vi "Button States Read.vi"(4 "error in (no error)":errorcluster, 6 "Container State":T3, 7 "Display State In":T1={"Buttons Displayed"=0, "Button States"=[], "Button Size"=0, "Button Style"=enum."Classic", "Active Button"=0, "Force Regen?"=FALSE, "Tip String Ref"=refnum}) -> (0 "error out":errorcluster, 2 "Value":bool[](array[boolean]), 3 "Display State Out":T1={"Buttons Displayed"=0, "Button States"=[], "Button Size"=0, "Button Style"=enum."Classic", "Active Button"=0, "Force Regen?"=FALSE, "Tip String Ref"=refnum})   [LabVIEW 2012, in "Toolbar.xctl"]
doc: "Read back which of the current buttons are in the 'on' state."
uses:
  Toolbar.xctl
  <vilib>/_xctls/Container State.ctl
  Toolbar State.ctl
  Button_Class/Button.lvclass
  Button_Class/Type Defs/Button Style.ctl
  Button_Class/Type Defs/Button Status.ctl
  <vilib>/_xctls/XControlSupport.lvlib
panel:
  # "Replace the Value Indicator below with an Indicator of desired type.\nDo not remove this Indicator or the others from the connector pane. \nDo not change the connector pane pattern.\nThe Value Indicator should always be the second terminal from top on the output side in the connector pane."
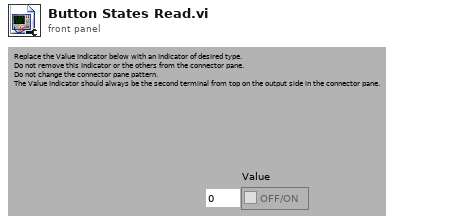
[diagram p1: front panel]
types:
  T1 = typedef "Toolbar.xctl/Toolbar State.ctl" = cluster{"Buttons Displayed":i32, "Button States":refnum<class "Button.lvclass">[], "Button Size":i32, "Button Style":T2, "Active Button":i32, "Force Regen?":bool, "Tip String Ref":refnum<vi>}
  T2 = typedef "Button.lvclass/Button Style.ctl" = enum16{"System", "Modern", "Classic", "Rounded", "Silver", "Ni Theme", "Metallic"}
  T3 = typedef "XControlSupport.lvlib/Container State.ctl" = cluster{"Indicator?":bool, "Run Mode?":bool, " Refnum":refnum<vi>}
  T4 = typedef "Button.lvclass/Button Status.ctl" = enum16{"Off", "Hover", "On", "Disabled"}
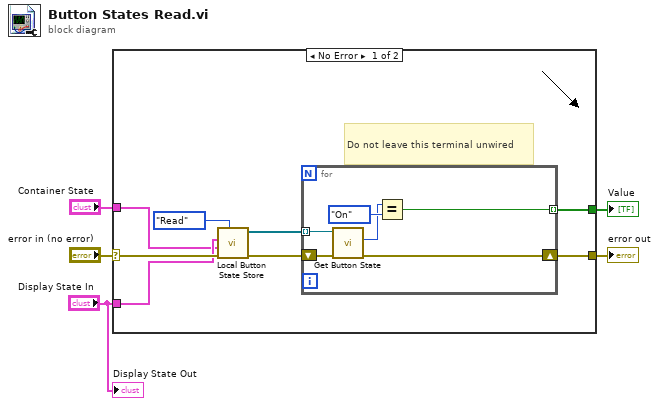
[diagram p0: block diagram]
diagram:
  n1 = case shown="No Error" "error in (no error)" {
    selector: "error in (no error)" -> [w11 w20]
    tunnel: [w13 _] -> w5
    tunnel: [w12 w20] -> w4
    tunnel: "Display State In" -> [w8 _]
    tunnel: "Container State" -> [w7 _]
    frame No Error {
      # "Do not leave this terminal unwired"
      n2 = call "Local Button State Store.vi"("Operation"=enum16{"Read", "Write"}."Read", "error in (no error)"=w11, "Container State"=w7, "Display State In"=w8) -> ("error out"=w10:errorcluster, "Button States"=w6:refnum<class "Button.lvclass">[])  [unwired: 6 out]
      n3 = for {
        tunnel: w6 -> [w17] mode=indexing
        tunnel: [w18] -> w13 mode=indexing
        shift-right: [w15] -> w12
        shift-left: w10 -> [w16]
        n4 = call-dynamic "Get Button State.vi"("error in (no error)"=w16, "Button in"=w17) -> ("error out"=w15:errorcluster, "State"=w14:T4)  [unwired: 8 out]
        n5 = Equal?(x=w14, y=Button_Status."On") -> (x = y?=w18:bool)
      }
    }
    frame Error {
    }
  }
  "error out" <- w4
  "Value" <- w5
  "Display State Out" <- "Display State In"
